vi "Set rect.vi"(8 "error in (no error)":errorcluster, 10 "rect":T1, 11 "Rectangle Border in":refnum<class "Rectangle Border.lvclass">) -> (0 "error out":errorcluster, 3 "Rectangle Border out":refnum<class "Rectangle Border.lvclass">)   [LabVIEW 2015, in "Rectangle Border.lvclass"]
uses:
  Rectangle Border.lvclass
  Rectangle Border.lvclass/Rectangle Border.ctl
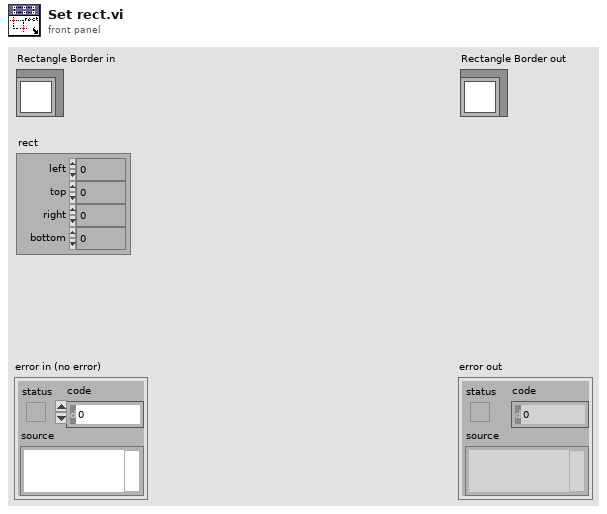
[diagram p1: front panel]
types:
  T1 = cluster{"left":i16, "top":i16, "right":i16, "bottom":i16}
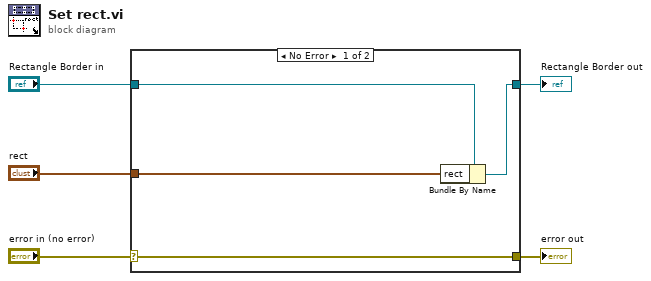
[diagram p0: block diagram]
diagram:
  n1 = case shown="No Error" "error in (no error)" {
    selector: "error in (no error)" -> [w9 w10]
    tunnel: [w9 w10] -> w4
    tunnel: [w7 w11] -> w2
    tunnel: "Rectangle Border in" -> [w8 w11]
    tunnel: "rect" -> [w6 _]
    frame No Error {
      n2 = Bundle By Name(cluster=w8, "rect"=w6) -> (w7:refnum<class "Rectangle Border.lvclass">)
    }
    frame Error {
    }
  }
  "error out" <- w4
  "Rectangle Border out" <- w2
